vi "REPORT_OPRTN_filter_columns.vi"(8 "error_in":errorcluster) -> (0 "error_out":errorcluster, 3 "Canceled?":bool=TRUE)   [LabVIEW 2019]
uses:
  FGV/REPORTS_records_display/FGV_REPORTS_records_display.ctl
  typedef/REPORT_OPRTN_all_info.ctl
  DATES/typedef/REPORT_DATES_statuses.ctl
  _misc/AULocalize/SubVIs/Get Localized Phrase Compact Interface 1D.vi
panel:
  in  "columns_filter":i32[](listbox)
  in  "ok":bool
  in  "cancel":bool
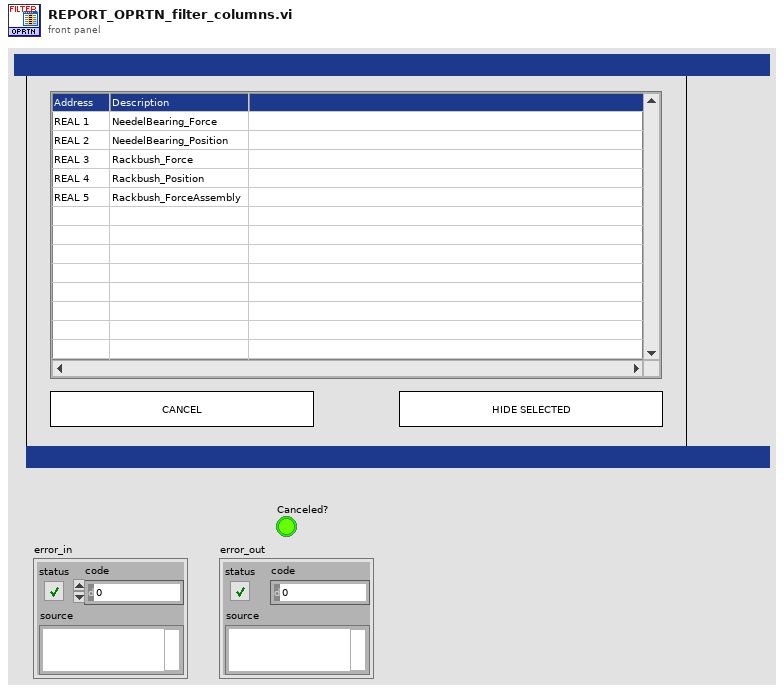
[diagram p1: front panel]
types:
  T1 = typedef "REPORT_OPRTN_all_info.ctl" = cluster{"OP":string, "date_start":string, "date_end":string, "time_start":string, "time_end":string, "filter_last_status":string, "no_of_static_columns":i32, "operations":string[][], "operations_statuses":T2[], "column_headers":string[], "archivisation_description":string[][], "displayed_rows":string[][], "displayed_statuses":T2[], "column_widths":i16[], "hidden_columns":i32[], "active_page":i32}
  T2 = typedef "REPORT_DATES_statuses.ctl" = enum16{"GEAR_OK", "GEAR_NOK", "GEAR_interrupted", "GEAR_in_operation", "GEAR_unexpected"}
  T3 = typedef "FGV_REPORTS_records_display.ctl" = enum16{"initialize", "GEAR_set_serial", "GEAR_set_header", "GEAR_set_operations", "GEAR_set_results", "GEAR_set_batches", "GEAR_get_serial", "GEAR_get_operation_IDs", "GEAR_toggle_results", "GEAR_show_all_results", "GEAR_hide_all_results", "GEAR_display", "GEAR_filter", "GEAR_restore", "GEAR_clear", "GEAR_get_all_info", "DATES_set_dates", "DATES_set_gears", "DATES_display", "DATES_filter", "DATES_first_page", "DATES_previous_page", "DATES_next_page", "DATES_last_page", "DATES_restore", "DATES_clear", "DATES_get_all_info", "PBATCH_set_batch_no", "PBATCH_set_gears", "PBATCH_display", "PBATCH_filter", "PBATCH_first_page", "PBATCH_previous_page", "PBATCH_next_page", "PBATCH_last_page", "PBATCH_restore", "PBATCH_clear", "PBATCH_get_all_info", "OPRTN_set_OP", "OPRTN_set_dates", "OPRTN_set_gears", "OPRTN_set_hidden_columns", "OPRTN_display", "OPRTN_filter", "OPRTN_filter_no_page_reset", "OPRTN_first_page", "OPRTN_previous_page", "OPRTN_next_page", "OPRTN_last_page", "OPRTN_restore", "OPRTN_clear", "OPRTN_get_all_info", "CFG_set_type", "CFG_set_dates", "CFG_set_records", "CFG_display", "CFG_filter", "CFG_first_page", "CFG_previous_page", "CFG_next_page", "CFG_last_page", "CFG_restore", "CFG_clear", "CFG_get_all_info", "AUDIT_set_dates", "AUDIT_set_records", "AUDIT_display", "AUDIT_filter", "AUDIT_first_page", "AUDIT_previous_page", "AUDIT_next_page", "AUDIT_last_page", "AUDIT_restore", "AUDIT_clear", "AUDIT_get_all_info", "OKNOK_set_dates", "OKNOK_set_records", "OKNOK_display", "OKNOK_restore", "OKNOK_clear", "OKNOK_get_all_info", "REWORKS_set_dates", "REWORKS_set_from_to", "REWORKS_set_records", "REWORKS_display", "REWORKS_filter", "REWORKS_first_page", "REWORKS_previous_page", "REWORKS_next_page", "REWORKS_last_page", "REWORKS_restore", "REWORKS_clear", "REWORKS_get_all_info", "PACE_set_dates", "PACE_set_limits", "PACE_set_records", "PACE_display", "PACE_restore", "PACE_clear", "PACE_get_all_info", "CBATCH_set_code", "CBATCH_set_records", "CBATCH_display", "CBATCH_filter", "CBATCH_first_page", "CBATCH_previous_page", "CBATCH_next_page", "CBATCH_last_page", "CBATCH_restore", "CBATCH_clear", "CBATCH_get_all_info", "CMPNT_set_serial", "CMPNT_set_records", "CMPNT_display", "CMPNT_first_page", "CMPNT_previous_page", "CMPNT_next_page", "CMPNT_last_page", "CMPNT_restore", "CMPNT_clear", "CMPNT_get_all_info", "clear"}
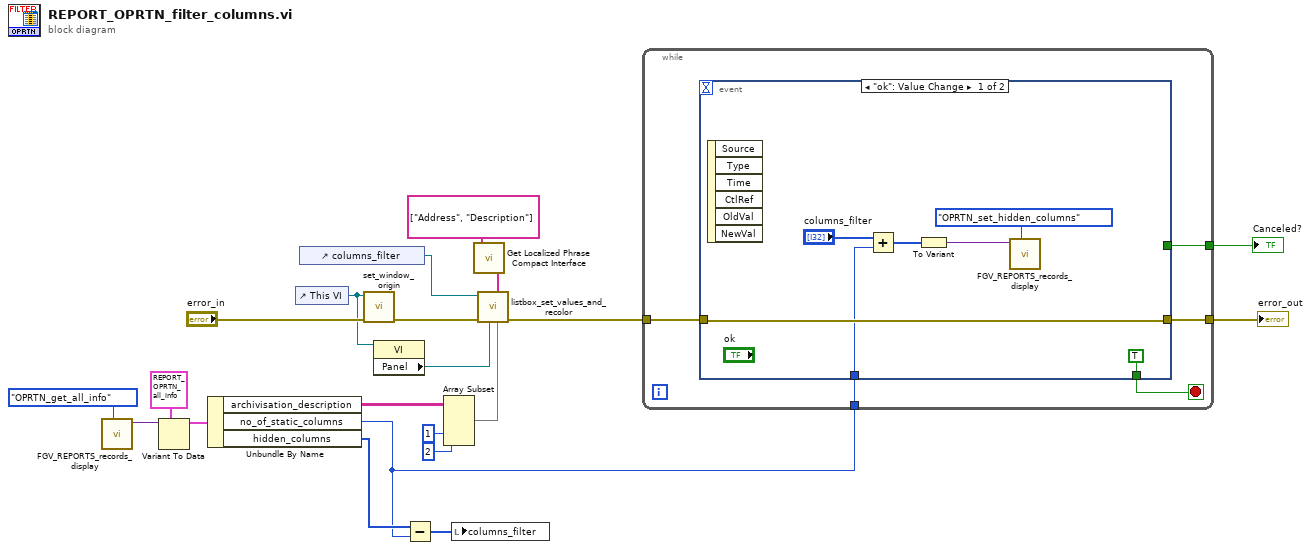
[diagram p0: block diagram]
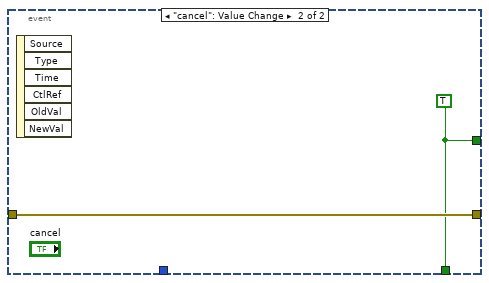
[diagram p2: hidden frame]
diagram:
  n1 = call "FGV_REPORTS_records_display.vi"("options"=FGV_REPORTS_records_display."OPRTN_get_all_info") -> ("output"=w17:variant)  [unwired: 9 in, 1 out]
  n2 = Variant To Data(type=T1 {"OP"="", "date_start"="", "date_end"="", "time_start"="", "time_end"="", "filter_last_status"="", "no_of_static_columns"=0, "operations"=[], "operations_statuses"=[], "column_headers"=[], "archivisation_description"=[], "displayed_rows"=[], "displayed_statuses"=[], "column_widths"=[], "hidden_columns"=[], "active_page"=0} ("REPORT_OPRTN_all_info"), Variant=w17) -> (data=w16:T1)  [unwired: 1 in, 1 out]
  n3 = Unbundle By Name(w16) -> ("archivisation_description"=w10:string[][], "no_of_static_columns"=w3:i32, "hidden_columns"=w4:i32[])
  n4 = control-ref of="This VI"() -> (w12:refnum<vi>)
  n5 = control-ref of="columns_filter"() -> (w13:refnum<vi>)
  n6 = call "set_window_origin.vi"("error_in"="error_in", "this_vi_reference"=w12) -> ("error_out"=w15:errorcluster)  [unwired: 9 in]
  n7 = property class="VI"(reference=w12) -> ("Panel"=w11:refnum<vi>)  [unwired: 1 in, 2 out]
  n8 = Subtract(x=w4, y=w3) -> (x-y=w2:i32[])
  n9 = Array Subset(array=w10, index (col)=1 ("index"), length (col)=2 ("length")) -> (w9:string[][])  [unwired: 2 in]
  n10 = local write "columns_filter"(w2) -> ()
  n11 = call-poly "Get Localized Phrase Compact Interface.vi"("Key"=string[] ["Address", "Description"] ("column_names")) -> ("Translated Phrase"=w1:string[])
  n12 = call "listbox_set_values_and_recolor.vi"("item_names"=w9, "front_panel_reference"=w11, "column_names"=w1, "error_in"=w15, "multicolumn_listbox_reference_in"=w13) -> ("error_out"=w14:errorcluster)  [unwired: 5 in, 1 out]
  n13 = while {
    tunnel: w14 -> [w26]
    tunnel: [w25] -> w21
    tunnel: w3 -> [w23]
    tunnel: [w22] -> w5
    stop <- w24 stop-if-true
    n14 = event shown="[0] \"ok\": Value Change" {
      selector: _ -> [_ _]
      dyn-events: _ -> [_ _]
      timeout: _ -> [_ _]
      tunnel: w26 -> [w33 w35]
      tunnel: [w33 w35] -> w25
      tunnel: [TRUE w34] -> w24
      tunnel: w23 -> [w31 _]
      tunnel: [_ w34] -> w22
      event "ok": Value Change {
        n15 = event-data() -> ()  [unwired: 1 in, 6 out]
        n16 = Add(x="columns_filter", y=w31) -> (x+y=w28:i32[])
        n17 = To Variant(anything=w28) -> (Variant=w27:variant)
        n18 = call "FGV_REPORTS_records_display.vi"("options"=FGV_REPORTS_records_display."OPRTN_set_hidden_columns", "input"=w27) -> ()  [unwired: 8 in, 2 out]
      }
      event "cancel": Value Change {
        w34 = TRUE
        n19 = event-data() -> ()  [unwired: 1 in, 6 out]
      }
    }
  }
  "error_out" <- w21
  "Canceled?" <- w5
